vi "Set_B.vi"(8 "error in (no error)":errorcluster, 9 "address string":string, 11 "Set Field (T)":dbl) -> (0 "error out":errorcluster)   [LabVIEW 2015]
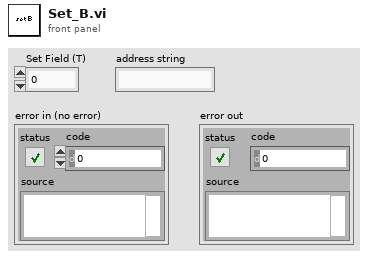
[diagram p1: front panel]
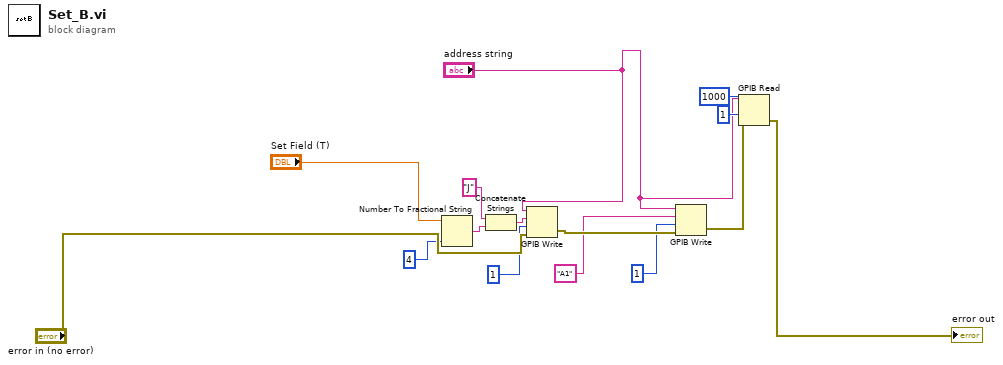
[diagram p0: block diagram]
diagram:
  n1 = Number To Fractional String(number="Set Field (T)", precision (6)=i16 4) -> (F-format string=w7:string)  [unwired: 2 in]
  n2 = Concatenate Strings("J" ("format string"), w7) -> (w8:string)
  n3 = GPIB Write(0:"address string", 1:w8, 2:i16 1 ("mode (0)"), 3:"error in (no error)") -> (6:w9:errorcluster)  [unwired: 1 in, 1 out]
  n4 = GPIB Write(0:"address string", 1:"A1" ("format string"), 2:i16 1 ("mode (0)"), 3:w9) -> (6:w11:errorcluster)  [unwired: 1 in, 1 out]
  n5 = GPIB Read(0:"address string", 1:1000 ("byte count"), 2:i16 1 ("mode (0)"), 3:w11) -> (7:→"error out":errorcluster)  [unwired: 1 in, 2 out]
